vi "check_whether_configuration_exists.vi"(8 "error in (no error)":errorcluster, 10 "configuration name":string, 11 "GenericPlugin in":refnum<class "ComponentTemplate.lvclass">) -> (0 "error out":errorcluster, 2 "exists?":bool, 3 "GenericPlugin out":refnum<class "ComponentTemplate.lvclass">)   [LabVIEW 2010]
uses:
  ComponentTemplate.lvclass
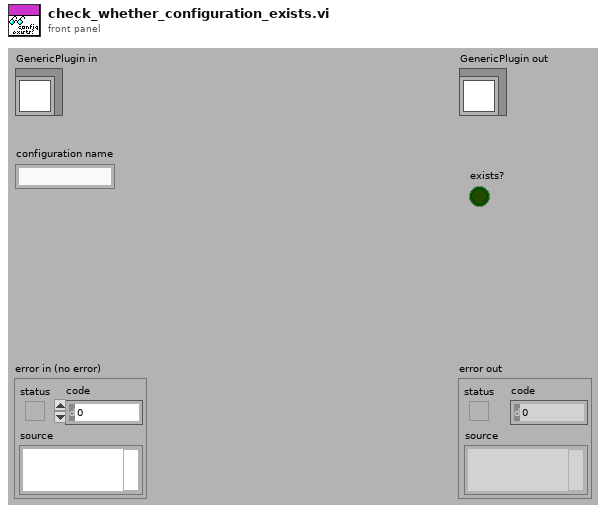
[diagram p1: front panel]
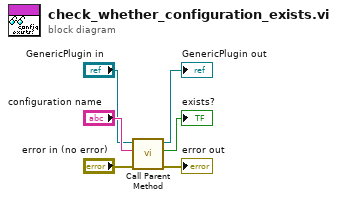
[diagram p0: block diagram]
diagram:
  n1 = call-parent "Call Parent Method"("error in (no error)"="error in (no error)", "configuration name"="configuration name", "GenericPlugin in"="GenericPlugin in") -> ("error out"=→"error out":errorcluster, "exists?"=→"exists?":bool, "GenericPlugin out"=→"GenericPlugin out":refnum<class "ComponentTemplate.lvclass">)  [unwired: 6 in]
